vi "Configure9203.vi"(7 "Channel Number":i32, 8 "error in (no error)":errorcluster, 10 "Properties":T1[](array[typedef]), 11 "IO Ref in":refnum<k21>) -> (0 "error out":errorcluster, 3 "IO Ref out":refnum<k21>)   [LabVIEW 2017, in "ScanEngine.lvlib"]
uses:
  <vilib>/addons/InsightCM/Devices/Shared/Common/ScanEngine/ScanEngine.lvlib
  <vilib>/addons/InsightCM/MessageBus/Base/controls/KeyValuePair.ctl
  <resource>/objmgr/cRIO.rc
  <vilib>/addons/InsightCM/Utilities/PropertyHelpers/PropertyHelpers.lvlib
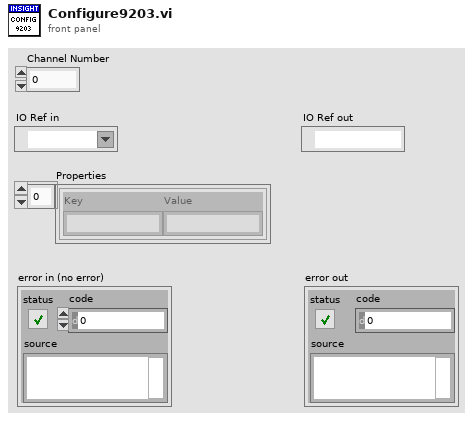
[diagram p1: front panel]
types:
  T1 = typedef "KeyValuePair.ctl" = cluster{"Key":string, "Value":string}
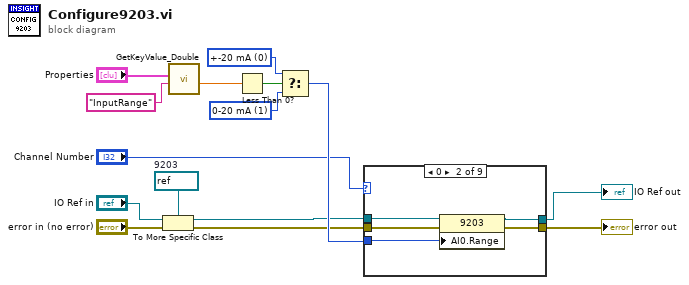
[diagram p0: block diagram]
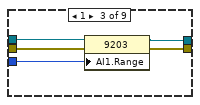
[diagram p3: hidden frame]
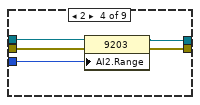
[diagram p4: hidden frame]
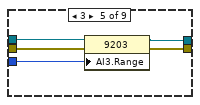
[diagram p5: hidden frame]
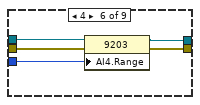
[diagram p6: hidden frame]
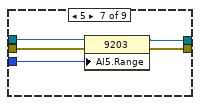
[diagram p7: hidden frame]
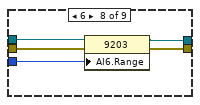
[diagram p8: hidden frame]
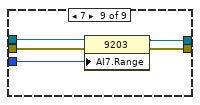
[diagram p9: hidden frame]
diagram:
  w11 = u32 1 items=["+-20 mA", "0-20 mA"] ("AI0:Range")
  w12 = u32 0 items=["+-20 mA", "0-20 mA"] ("AI0:Range")
  w6 = refnum<k21> refnum  # 9203
  n1 = To More Specific Class(target class=w6, reference="IO Ref in", error in="error in (no error)") -> (specific class reference=w8:refnum<k21>, error out=w14:errorcluster)
  n2 = call <vilib>:"GetKeyValue_Double.vi"("key"="InputRange" ("name"), "key value pairs"="Properties") -> ("value"=w1:dbl)  [unwired: 7 in, 2 out]
  n3 = Less Than 0?(x=w1) -> (x < 0?=w13:bool)
  n4 = Select(t=w12, s=w13, f=w11) -> (s? t:f=w15:u32)
  n5 = case shown="0" "Channel Number" {
    tunnel: w8 -> [w17 w22 w27 w32 w37 w42 w47 w52 w57]
    tunnel: w14 -> [w16 w21 w26 w31 w36 w41 w46 w51 w56]
    tunnel: [w17 w20 w25 w30 w35 w40 w45 w50 w55] -> w9
    tunnel: [w16 w19 w24 w29 w34 w39 w44 w49 w54] -> w10
    tunnel: w15 -> [_ w18 w23 w28 w33 w38 w43 w48 w53]
    frame -1, Default {
    }
    frame 0 {
      n6 = property class="9203"(reference=w22, error in=w21, "AI0.Range"=w18) -> (reference out=w20:refnum<k21>, error out=w19:errorcluster)
    }
    frame 1 {
      n7 = property class="9203"(reference=w27, error in=w26, "AI1.Range"=w23) -> (reference out=w25:refnum<k21>, error out=w24:errorcluster)
    }
    frame 2 {
      n8 = property class="9203"(reference=w32, error in=w31, "AI2.Range"=w28) -> (reference out=w30:refnum<k21>, error out=w29:errorcluster)
    }
    frame 3 {
      n9 = property class="9203"(reference=w37, error in=w36, "AI3.Range"=w33) -> (reference out=w35:refnum<k21>, error out=w34:errorcluster)
    }
    frame 4 {
      n10 = property class="9203"(reference=w42, error in=w41, "AI4.Range"=w38) -> (reference out=w40:refnum<k21>, error out=w39:errorcluster)
    }
    frame 5 {
      n11 = property class="9203"(reference=w47, error in=w46, "AI5.Range"=w43) -> (reference out=w45:refnum<k21>, error out=w44:errorcluster)
    }
    frame 6 {
      n12 = property class="9203"(reference=w52, error in=w51, "AI6.Range"=w48) -> (reference out=w50:refnum<k21>, error out=w49:errorcluster)
    }
    frame 7 {
      n13 = property class="9203"(reference=w57, error in=w56, "AI7.Range"=w53) -> (reference out=w55:refnum<k21>, error out=w54:errorcluster)
    }
  }
  "error out" <- w10
  "IO Ref out" <- w9
